vi "FTW-TestExecutive-Core_StepType_ConfigClass.vi"(0 "Step Class":refnum<class "FTW-TestStep-Base.lvclass">, 1 "Other Config Items":string="{}", 5 "Inbox Address":string) -> (4 "Base Config String":string="{}")   [LabVIEW 2015, in "FTW-TestExecutive-Core.lvclass"]
uses:
  FTW-TestExecutive-Core.lvclass
  Test Steps/Base/FTW-TestStep-Base.lvclass
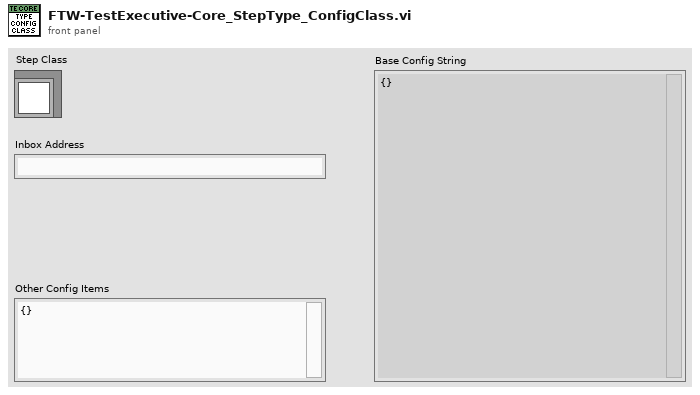
[diagram p1: front panel]
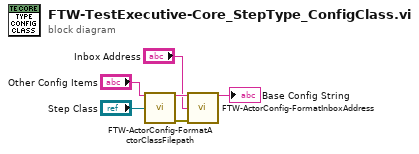
[diagram p0: block diagram]
diagram:
  n1 = call "FTW-ActorConfig-FormatActorClassFilepath.vi"("FTW Config String In"="Other Config Items", "Actor Instance"="Step Class") -> ("FTW Config String"=w5:string, "error out"=w4:errorcluster)  [unwired: 12 in]
  n2 = call "FTW-ActorConfig-FormatInboxAddress.vi"("FTW Config String In"=w5, "Inbox Address"="Inbox Address", "error in"=w4) -> ("FTW Config String"=→"Base Config String":string)  [unwired: 11 in, 1 out]
